vi "FCS16.vi"(11 "Input string":string) -> (3 "hex integer string":string)   [LabVIEW 2020]
uses:
  DLL_FCS proj.dll
panel:
  out "unsigned byte array":u8[](array[numeric])
  out "return type":u16
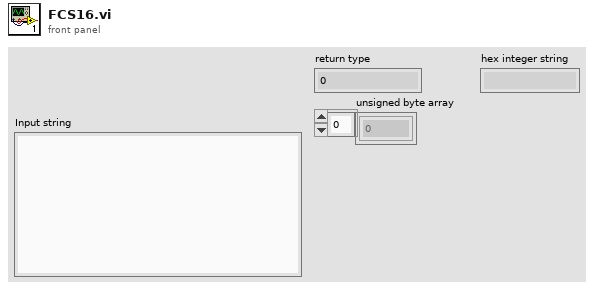
[diagram p1: front panel]
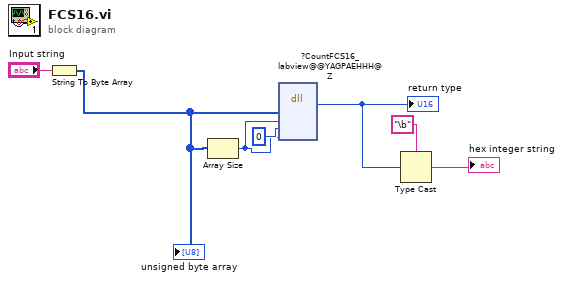
[diagram p0: block diagram]
diagram:
  n1 = String To Byte Array(string="Input string") -> (unsigned byte array=w5:u8[])
  "unsigned byte array" <- w5
  n2 = Array Size(array=w5) -> (size(s)=w4:i32)
  n3 = dll-call lib="H:/USB/KTC/Instrument/Electricity center/Electricity meter_DLMS/Subvi/DLL_FCS proj.dll" fn="?CountFCS16_labview@@YAGPAEHHH@Z"("input array"=w5, "array_size"=w4, "index"=0, "count"=w4) -> ("return type"=w3:u16)  [unwired: 7 in, 2 out]
  "return type" <- w3
  n4 = Type Cast(type="\b", x=w3) -> (*(type *) &x=→"hex integer string":string)
